vi "AFT Filter Signal.vi"   [LabVIEW 2017, in "NI_AdaptiveFilter.lvlib"]
doc: "Filters an input signal with an adaptive filter point by point. You must use the least mean squares (LMS) or recursive least squares (RLS) algorithms to create the adaptive filter. Unlike the AFT Filter Signal and Update Coefficients VI, the AFT Filter Signal VI does not update the coefficients of the adaptive filter. Use the AFT Update Coefficients VI to update the filter coefficients. Wire data to the <B>x(n)</B> input to determine the polymorphic instance to use or manually select the instance. The data type of the adaptive filter that you wire to the <B>adaptive filter in</B> input must match the instance of the AFT Filter Signal VI."
uses:
  <vilib>/addons/Adaptive Filters/NI_AdaptiveFilter.lvlib
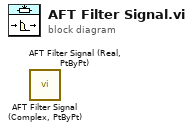
[diagram p0: block diagram]
diagram:
  n1 = call <vilib>:"AFT Filter Signal (Complex, PtByPt).vi"() -> ()  [unwired: 9 in, 3 out]
  n2 = call <vilib>:"AFT Filter Signal (Real, PtByPt).vi"() -> ()  [unwired: 9 in, 3 out]
